vi "invoke method.vi"   [LabVIEW 2013, in "call function by reference.lvclass"]
uses:
  call function by reference.lvclass
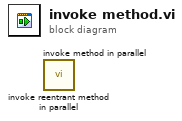
[diagram p0: block diagram]
diagram:
  n1 = call "invoke reentrant method in parallel.vi"() -> ()  [unwired: 10 in, 2 out]
  n2 = call "invoke method in parallel.vi"() -> ()  [unwired: 10 in, 2 out]
